vi "sub_Gen_Sync_Params.vi"(7 "IQ Sampling\nRate [s/sec]":dbl, 8 "Packet Parameters in":T1={"Length of sync sequence (50)"=50, "Number of message bits"=128, "Number of guardbits"=40, "Sync PN sequence order (31)"=31, "Number of header bits"=16, "Packet Pad [samples]"=0}, 9 "matched filter coefficients":dbl[](array[numeric]) format="%^.2e", 10 "pulse shaping filter coefficients":dbl[](array[numeric]) format="%.2f", 11 "QPSK System Parameters in":T2={"Samples per Symbol"=8, "symbol map"=[], "Differential PSK"=enum."disable", "PSK type"=0, "M-PSK"=4} caption="QPSK System Parameters" {"PSK type" items=["normal", "shifted", "offset"]; "symbol map" format="%.3f"}) -> (0 "Payload length":i32, 1 "Frame Length (samples)":i32, 2 "Expected Xcorr Index":i32, 3 "Sync Sequence Waveform":cdb[](array[numeric]), 4 "Sync Sequence Bitstream":i8[](array[numeric]))   [LabVIEW 2014]
uses:
  <vilib>/addons/Modulation/Digital/General/MT Generate Bits (Galois, PN Order).vi
  <vilib>/Analysis/2dsp.llb/1D Cross Correlation (CDB).vi
  <vilib>/addons/Modulation/Digital/Support/Common/Validators/mod_Generate Bits Validate.vi
  <vilib>/addons/Modulation/Analog/support/mod_Set Error Source.vi
  <vilib>/addons/Modulation/Digital/General/MT Generate PSK System Parameters(M).vi
  <vilib>/addons/Modulation/Digital/General/subVIs/mod_Generate Bits PN Sequence.vi
  <vilib>/addons/Modulation/Digital/General/MT Apply Matched Filter (Generic).vi
  <vilib>/Analysis/NI_AALPro.lvlib
  <vilib>/addons/Modulation/niDMT.lvlib
panel:
  out "max value 2":dbl
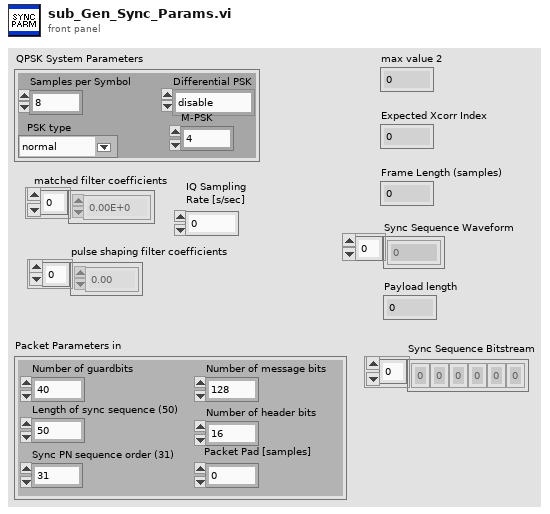
[diagram p1: front panel]
types:
  T1 = cluster{"Length of sync sequence (50)":i32, "Number of message bits":i32, "Number of guardbits":i32, "Sync PN sequence order (31)":i32, "Number of header bits":i32, "Packet Pad [samples]":i32}
  T2 = cluster{"Samples per Symbol":i32, "symbol map":cdb[], "Differential PSK":enum16{"disable", "enable"}, "PSK type":u16, "M-PSK":i32}
  T3 = cluster{"samples per symbol (16)":i32, "symbol map":cdb[], "differential PSK":enum16{"disable", "enable"}, "PSK type":u16}
  T4 = typedef "niAMT.lvlib/Complex Data Waveform.ctl" = cluster{"t0":dbl, "dt":dbl, "Y":cdb[]}
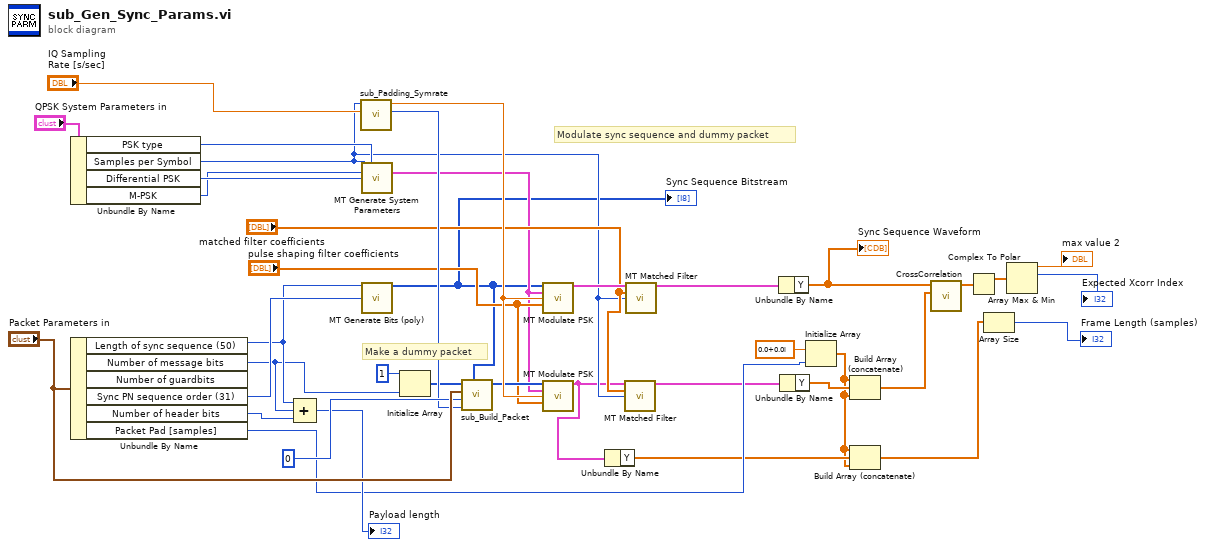
[diagram p0: block diagram]
diagram:
  # "Make a dummy packet"
  # "Modulate sync sequence and dummy packet"
  n1 = Unbundle By Name("QPSK System Parameters in") -> ("PSK type"=w38:u16, "Samples per Symbol"=w11:i32, "Differential PSK"=w36:enum16{"disable", "enable"}, "M-PSK"=w23:i32)
  n2 = Unbundle By Name("Packet Parameters in") -> ("Length of sync sequence (50)"=w22:i32, "Number of message bits"=w21:i32, "Sync PN sequence order (31)"=w39:i32, "Number of header bits"=w20:i32, "Packet Pad [samples]"=w14:i32)  [unwired: 1 out]
  n3 = Compound Arithmetic op=ADD(w22, w21, w20) -> (→"Payload length":i32)
  n4 = call "sub_Padding_Symrate.vi"("Tx IQ Sampling\nRate [s/sec]"="IQ Sampling\nRate [s/sec]", "Samples per Symbol"=w11) -> ("Padding Bits"=w27:i32, "Symbol Rate"=w30:dbl)  [unwired: 8 in]
  n5 = call-poly <vilib>:"MT Generate System Parameters.vi"("samples per symbol (16)"=w11, "PSK type"=w38, "M-PSK (4)"=w23, "differential PSK"=w36) -> ("PSK system parameters"=w6:T3)  [unwired: 9 in, 2 out]
  n6 = call-poly <vilib>:"MT Generate Bits (poly).vi"("total bits (128)"=w22, "PN sequence order (9)"=w39) -> ("output bit stream"=w1:i8[])  [unwired: 11 in, 2 out]
  "Sync Sequence Bitstream" <- w1
  n7 = Initialize Array(i8 1, w21) -> (w25:i8[])
  n8 = call "sub_Build_Packet.vi"("Sync Sequence Bitstream"=w1, "Cyclic Padding Bits"=w27, "Packet number"=i16 0, "Packet Parameters in"="Packet Parameters in", "Input Message"=w25) -> ("Packet out"=w24:i8[])  [unwired: 6 in]
  n9 = call <vilib>:"MT Modulate PSK.vi"("input bit stream"=w1, "PSK system parameters"=w6, "symbol rate (Hz)"=w30, "pulse shaping filter coefficients"="pulse shaping filter coefficients") -> ("output complex waveform"=w13:T4)  [unwired: 9 in, 2 out]
  n10 = call <vilib>:"MT Modulate PSK.vi"("input bit stream"=w24, "PSK system parameters"=w6, "symbol rate (Hz)"=w30, "pulse shaping filter coefficients"="pulse shaping filter coefficients") -> ("output complex waveform"=w5:T4)  [unwired: 9 in, 2 out]
  n11 = Unbundle By Name(w5) -> ("Y"=w4:cdb[])
  n12 = call-poly <vilib>:"MT Matched Filter.vi"("input complex waveform"=w5, "matched filter coefficients"="matched filter coefficients", "samples per symbol (16)"=w11) -> ("output complex waveform"=w9:T4)  [unwired: 11 in, 1 out]
  n13 = call-poly <vilib>:"MT Matched Filter.vi"("input complex waveform"=w13, "matched filter coefficients"="matched filter coefficients", "samples per symbol (16)"=w11) -> ("output complex waveform"=w10:T4)  [unwired: 11 in, 1 out]
  n14 = Unbundle By Name(w10) -> ("Y"=w33:cdb[])
  "Sync Sequence Waveform" <- w33
  n15 = Unbundle By Name(w9) -> ("Y"=w16:cdb[])
  n16 = Initialize Array(cdb 0.0+0.0i ("element"), w14) -> (w2:cdb[])
  n17 = Build Array (concatenate)(w2, w16, w2) -> (w15:cdb[])
  n18 = Build Array (concatenate)(w2, w4, w2) -> (w3:cdb[])
  n19 = call-poly <vilib>:"CrossCorrelation.vi"("Y"=w15, "X"=w33) -> ("Rxy"=w8:cdb[])  [unwired: 8 in, 1 out]
  n20 = Complex To Polar(r * e^(i*theta)=w8) -> (r=w7:dbl[])  [unwired: 1 out]
  n21 = Array Size(array=w3) -> (size(s)=→"Frame Length (samples)":i32)
  n22 = Array Max & Min(array=w7) -> (max value=→"max value 2":dbl, max index (indices)=→"Expected Xcorr Index":i32)  [unwired: 2 out]
